vi "C_Init.vi"(8 "error in (no error)":errorcluster, 11 "Object in":refnum<class "C.lvclass">) -> (0 "error out":errorcluster, 3 "object out":refnum<class "C.lvclass">)   [LabVIEW 2013, in "C.lvclass"]
uses:
  C.lvclass
  C.lvclass/C.ctl
  B_class/B.lvclass
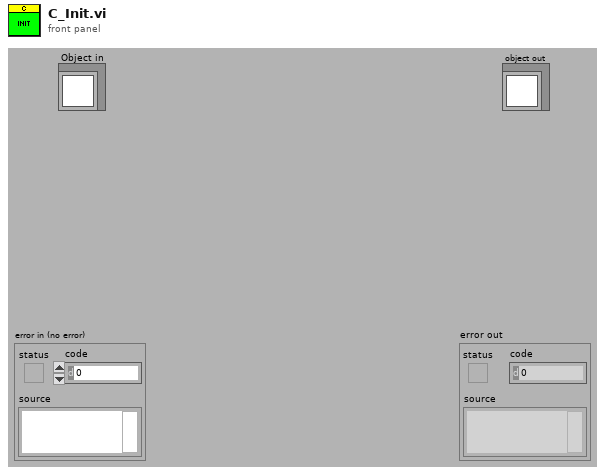
[diagram p1: front panel]
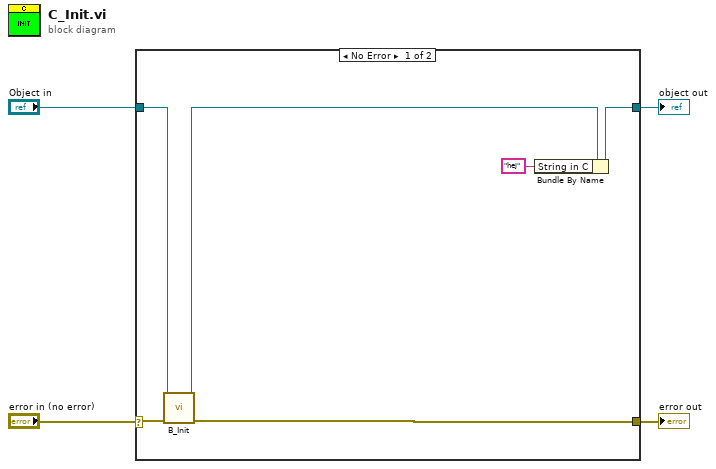
[diagram p0: block diagram]
diagram:
  n1 = case shown="No Error" "error in (no error)" {
    selector: "error in (no error)" -> [w9 w11]
    tunnel: [w10 w12] -> w4
    tunnel: "Object in" -> [w7 w12]
    tunnel: [w8 w11] -> w1
    frame No Error {
      n2 = call "B_Init.vi"("error in (no error)"=w9, "object in"=w7) -> ("error out"=w8:errorcluster, "object out"=w6:refnum<class "C.lvclass">)  [unwired: 8 in]
      n3 = Bundle By Name(cluster=w6, "String in C"="hej") -> (w10:refnum<class "C.lvclass">)
    }
    frame Error {
    }
  }
  "object out" <- w4
  "error out" <- w1
